vi "Host_PulseHistogram_OnlyLaser.vi"() -> ()   [LabVIEW 2012]
uses:
  <vilib>/FPGAPlugInAG/PXIe-7962R/niLvFpga_Open_PXIe-7962R.vi
  <vilib>/rvi/interface/common/dynamic/niFpgaDynamicAddResources.vi
  <vilib>/Utility/error.llb/Error Cluster From Error Code.vi
  <vilib>/rvi/errors/niLvFpgaAdjustHostInterfaceError.vi
  <vilib>/FPGAPlugInAG/Dynamic/niLvFpga_Close_Dynamic.vi
  <vilib>/rvi/interface/nirviOpenFPGA/nirviOpenFPGA.xnode
  FPGA Bitfiles/PulseHistogram_OnlyLaser_PXIe-7962R.lvbitx
  <vilib>/rvi/interface/nirviReadWriteControl/nirviReadWriteControl.xnode
  <vilib>/rvi/interface/nirviMethod/nirviMethod.xnode
  <vilib>/rvi/interface/nirviCloseFPGA/nirviCloseFPGA.xnode
  <vilib>/rvi/interface/Simulation/niFpgaSimulationCallBeginRW.vi
  NiFpgaLv.dll
  <vilib>/FPGAPlugInAG/Dynamic/niLvFpga_ReadFifo_Dynamic.vi
  <vilib>/rvi/errors/niLvFpgaMergeErrorWithErrorCode.vi
panel:
  out "Interflank intervals":i32[](graph)
  out "Loop counter":i32
  out "Waveform Graph":waveform(i16)(graph)
  out "Interloop FIFO timed out":bool
  out "Acq FIFO overflow":bool
  out "Interloop FIFO overflow":bool
  out "Reference pulse frequency":dbl format="%#_5p"
  out "Total sample count":u64
  out "Total reference pulse count":u64
  out "Reference pulse length histogram":T1(graph)
  out "Reference pulse period histogram":T1(graph)
  out "Sampling frequency":dbl format="%#_6p"
  out "Sampling interval":dbl format="%#_6p"
  in  "Onboard clock frequency":dbl=500000000.0 format="%#_6p"
  in  "Quit":bool
  # "Set clock before start!"
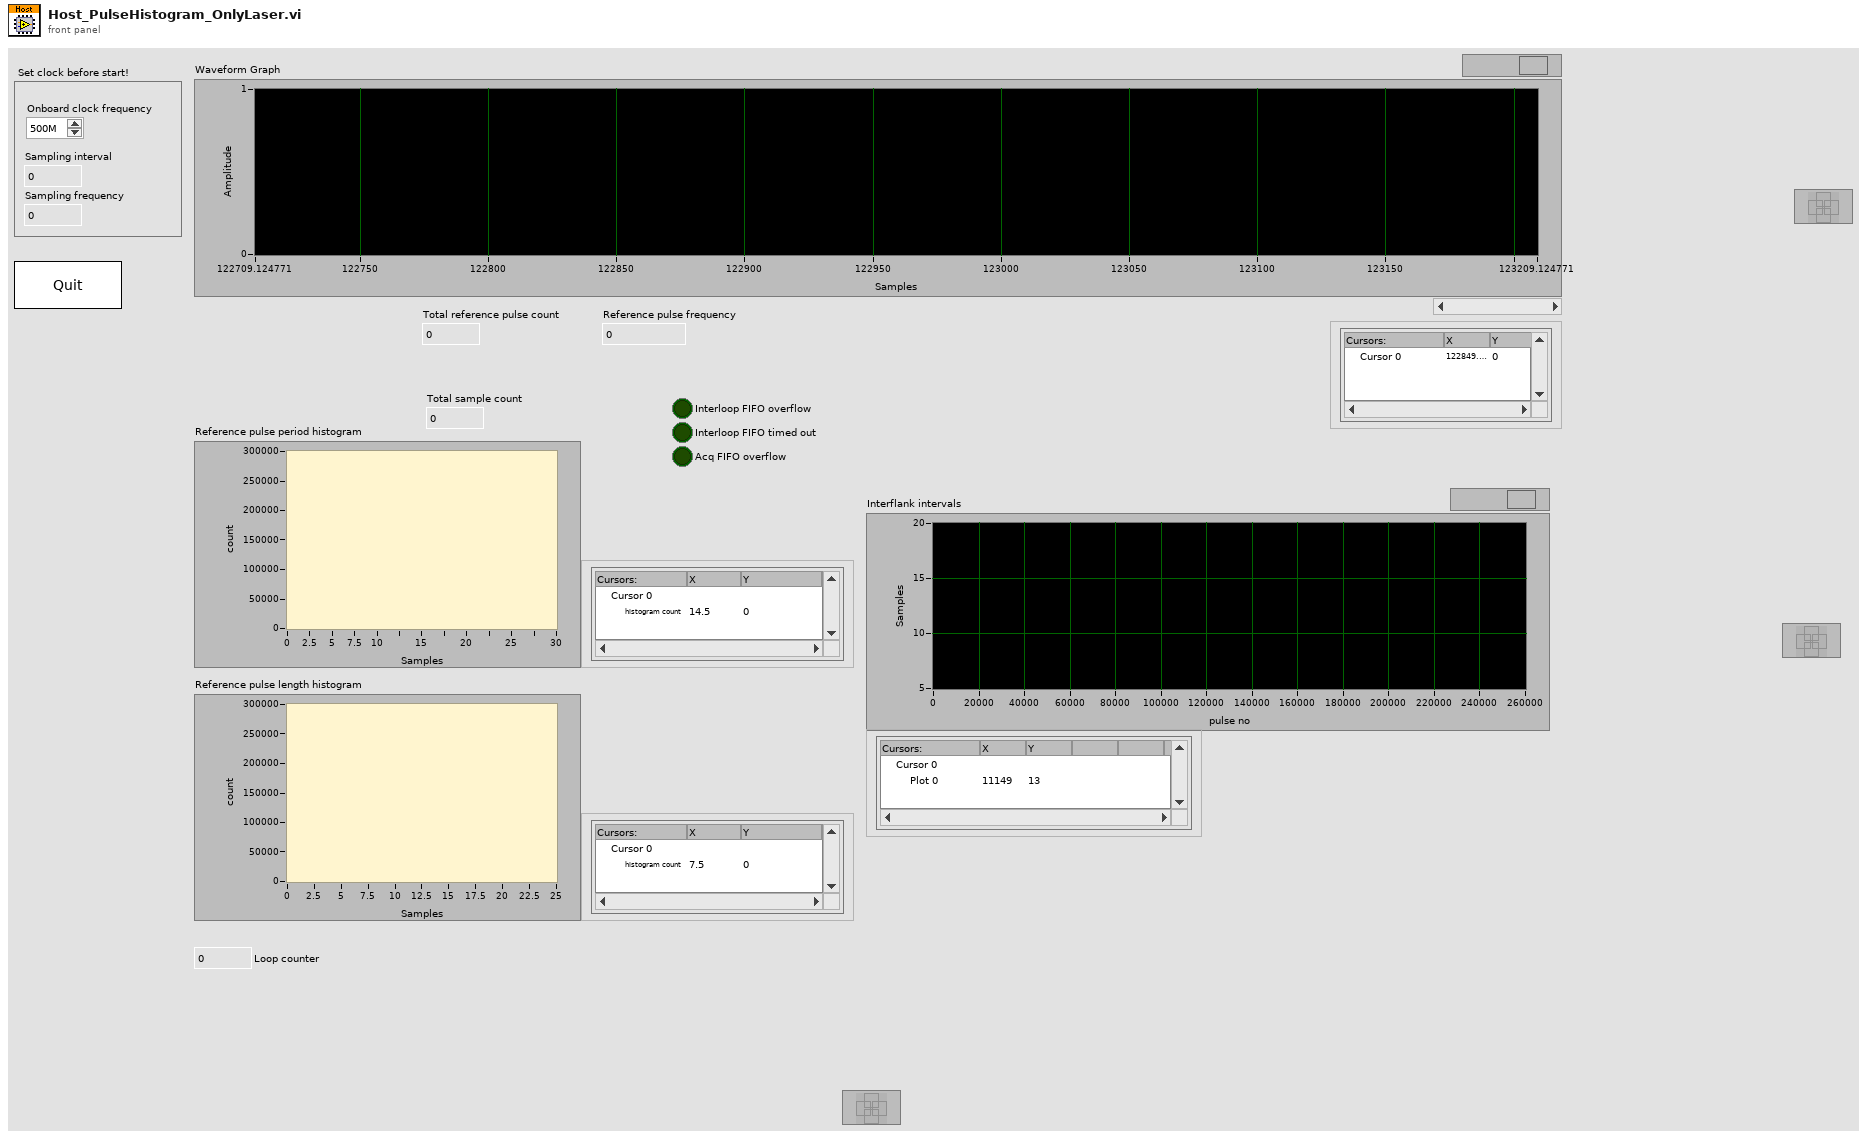
[diagram p1: front panel]
types:
  T1 = cluster{"X Values":dbl[], "Histogram: h(x)":i32[]}
  T2 = enum8{"Enabled", "Disabled", "Disabled and Grayed Out"}
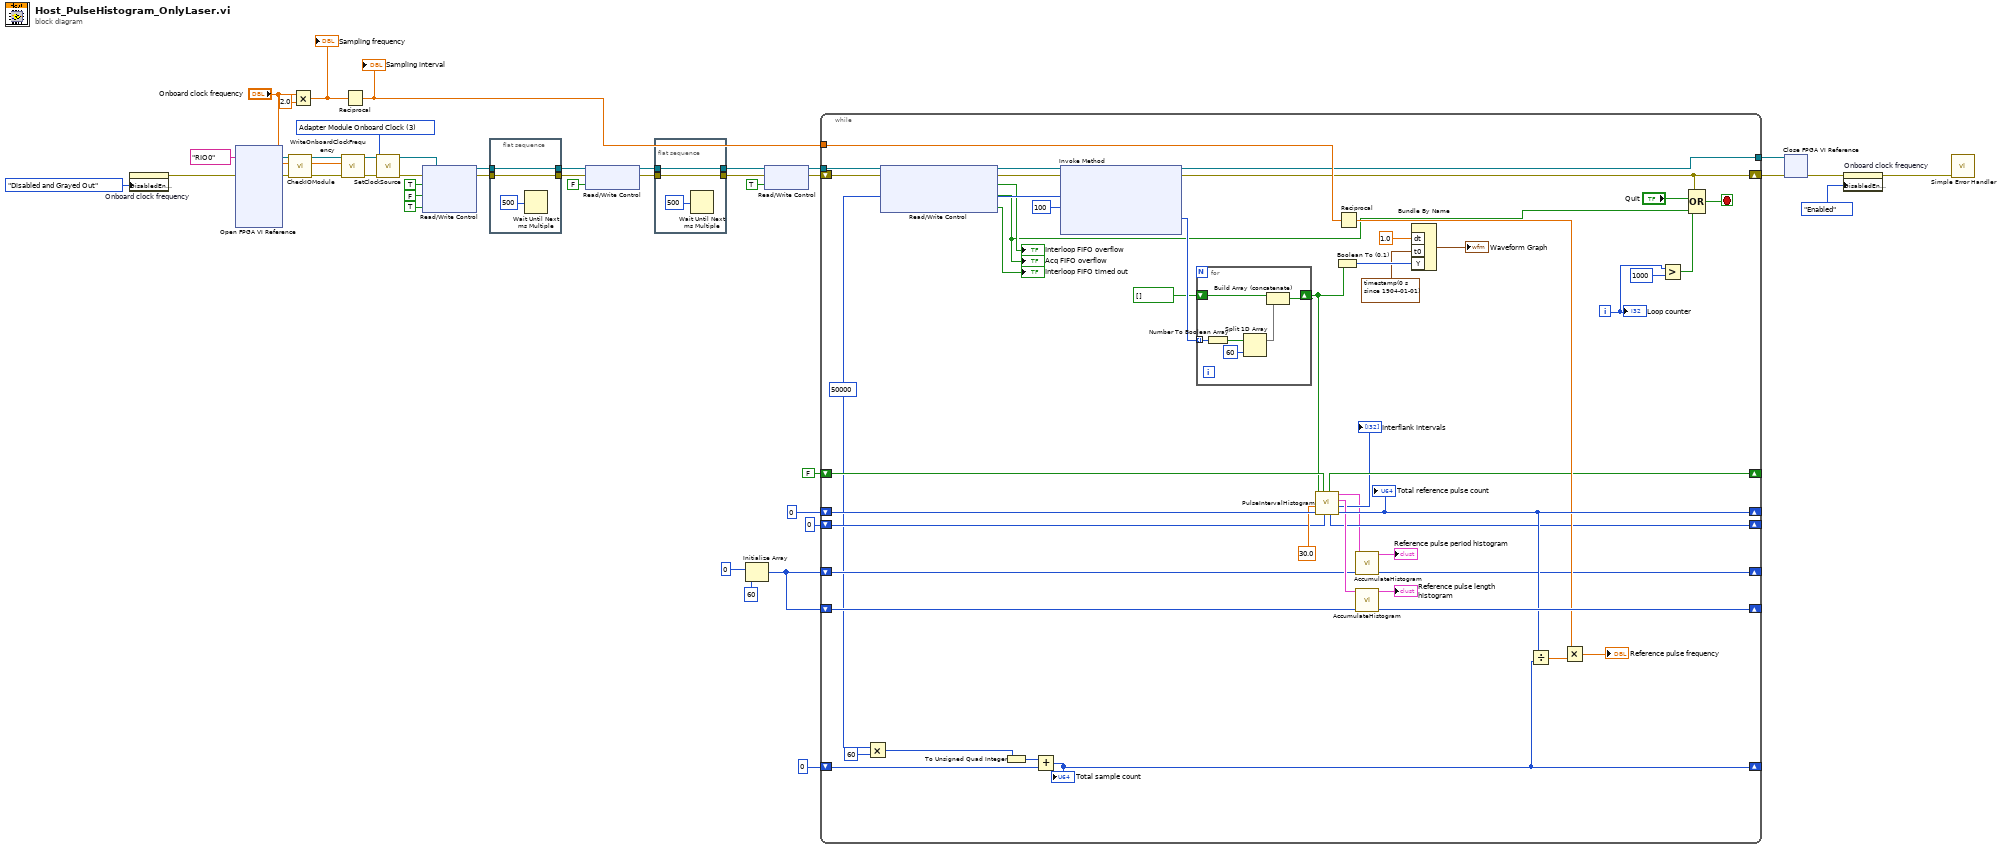
[diagram p0: block diagram]
diagram:
  w43 = u8 3 items=["Tristate"=0, "Sync Clock (PXIe only)"=2, "Adapter Module Onboard Clock"=3, "Strobe from Crosspoint Switch"=4, "Strobe Bypass"=5] ("Clock Source")
  n1 = property on="Onboard clock frequency" class="DigNum (strict)"("DisabledEnum"=T2."Disabled and Grayed Out" ("Disabled")) -> (error out=w27:errorcluster)  [unwired: 2 in, 1 out]
  n2 = xnode "Open FPGA VI Reference"("error in"=w27, "resource name"=tag "RIO0") -> ("FPGA VI Reference Out"=w7:refnum<k20>, "error out"=w6:errorcluster)
  n3 = call "CheckIOModule.vi"("error in (no error)"=w6, "FPGA VI Reference In"=w7) -> ("error out"=w37:errorcluster, "FPGA VI Reference Out"=w36:refnum<k20>)  [unwired: 8 in]
  n4 = Multiply(x="Onboard clock frequency", y=2.0) -> (x*y=w31:dbl)
  "Sampling frequency" <- w31
  n5 = call "WriteOnboardClockFrequency.vi"("error in (no error)"=w37, "Onboard clock frequency"="Onboard clock frequency", "FPGA VI Reference In"=w36) -> ("error out"=w35:errorcluster, "FPGA VI Reference Out"=w34:refnum<k20>)  [unwired: 7 in]
  n6 = Reciprocal(x=w31) -> (1/x=w30:dbl)
  "Sampling interval" <- w30
  n7 = call "SetClockSource.vi"("error in (no error)"=w35, "Clock Source"=w43, "FPGA VI Reference In"=w34) -> ("error out"=w41:errorcluster, "FPGA VI Reference Out"=w42:refnum<k20>)  [unwired: 7 in]
  n8 = xnode "Read/Write Control"("FPGA VI Reference In"=w42, "error in"=w41, "Commit"=TRUE, "Acq_Reset"=FALSE, "Acq_Reset"=TRUE) -> ("FPGA VI Reference Out"=w17:refnum<k20>, "error out"=w16:errorcluster)
  n9 = flat-sequence {
    tunnel: w17 -> [w44]
    tunnel: w16 -> [w45]
    tunnel: [w45] -> w14
    tunnel: [w44] -> w15
    frame #0 {
      n10 = Wait Until Next ms Multiple(millisecond multiple=u32 500) -> ()  [unwired: 1 out]
    }
  }
  n11 = xnode "Read/Write Control"("FPGA VI Reference In"=w15, "error in"=w14, "Acq_Reset"=FALSE) -> ("FPGA VI Reference Out"=w9:refnum<k20>, "error out"=w8:errorcluster)
  n12 = flat-sequence {
    tunnel: w9 -> [w47]
    tunnel: w8 -> [w48]
    tunnel: [w48] -> w4
    tunnel: [w47] -> w5
    frame #0 {
      n13 = Wait Until Next ms Multiple(millisecond multiple=u32 500) -> ()  [unwired: 1 out]
    }
  }
  n14 = Initialize Array(0, 60 ("dimension size")) -> (w19:i32[])
  n15 = xnode "Read/Write Control"("FPGA VI Reference In"=w5, "error in"=w4, "Acquire"=TRUE) -> ("FPGA VI Reference Out"=w3:refnum<k20>, "error out"=w2:errorcluster)
  n16 = while {
    tunnel: w3 -> [w54]
    tunnel: w30 -> [w82]
    shift-right: [w57] -> w29
    shift-left: w2 -> [w53]
    tunnel: [w58] -> w28
    shift-right: [w73] -> _
    shift-left: w19 -> [w63]
    shift-right: [w97] -> _
    shift-left: w19 -> [w96]
    shift-right: [w95] -> _
    shift-left: u64 0 ("Pulse count out") -> [w94]
    shift-right: [w69] -> _
    shift-left: u64 0 ("Pulse count out") -> [w93]
    shift-right: [w77] -> _
    shift-left: FALSE ("Last reference value out") -> [w76]
    shift-right: [w75] -> _
    shift-left: 0 ("Last rising flank out") -> [w74]
    i -> [w65]
    stop <- w72 stop-if-true
    w59 = u32 50000 ("Number of Elements")
    n17 = Multiply(x=w59, y=u32 60) -> (x*y=w84:u32)
    n18 = xnode "Read/Write Control"("FPGA VI Reference In"=w54, "error in"=w53) -> ("FPGA VI Reference Out"=w51:refnum<k20>, "error out"=w52:errorcluster, "Interloop FIFO overflow"=→"Interloop FIFO overflow":bool, "ToHostLaserFIFO overflow"=w50:bool, "Interloop FIFO timed out"=→"Interloop FIFO timed out":bool)
    "Acq FIFO overflow" <- w50
    n19 = To Unsigned Quad Integer(1:w84) -> (0:w83:u64)
    n20 = Add(x=w83, y=w93) -> (x+y=w69:u64)
    "Total sample count" <- w69
    n21 = xnode "Invoke Method"("FPGA VI Reference In"=w51, "error in"=w52, "Number of Elements"=w59, "Timeout (ms)"=100) -> ("FPGA VI Reference Out"=w58:refnum<k20>, "error out"=w57:errorcluster, "Data"=w86:u64[])  [unwired: 1 out]
    n22 = for {
      tunnel: w86 -> [w102] mode=indexing
      shift-right: [w100] -> w61
      shift-left: bool[] [] -> [w99]
      n23 = Number To Boolean Array(number=w102) -> (Boolean array=w103:bool[])
      n24 = Split 1D Array(array=w103, index=60) -> (first subarray=w98:bool[])  [unwired: 1 out]
      n25 = Build Array (concatenate)(w99, w98) -> (w100:bool[])
    }
    n26 = call "PulseIntervalHistogram.vi"("Last rising flank in"=w74, "Last reference value in"=w76, "Pulse count in"=w94, "No of SI bins"=30.0, "Binary array probe"=w61) -> ("Pulse count out"=w95:u64, "Interflank intervals out"=→"Interflank intervals":i32[], "Pulse length histogram"=w90:T1, "Pulse period histogram"=w64:T1, "Last rising flank out"=w75:i32, "Last reference value out"=w77:bool)  [unwired: 1 in]
    "Total reference pulse count" <- w95
    n27 = Boolean To (0,1)(Boolean=w61) -> (0, 1=w92:i16[])
    n28 = Reciprocal(x=w82) -> (1/x=w80:dbl)
    n29 = call "AccumulateHistogram.vi"("Array in"=w63, "Histogram graph in"=w64) -> ("Array out"=w73:i32[], "Histogram graph out"=→"Reference pulse period histogram":T1)  [unwired: 8 in]
    n30 = call "AccumulateHistogram.vi"("Array in"=w96, "Histogram graph in"=w90) -> ("Array out"=w97:i32[], "Histogram graph out"=→"Reference pulse length histogram":T1)  [unwired: 8 in]
    n31 = Bundle By Name("dt"=1.0, "t0"=timestamp(0 s since 1904-01-01), "Y"=w92) -> (→"Waveform Graph":waveform(i16))  [unwired: 1 in]
    n32 = Divide(x=w95, y=w69) -> (x/y=w87:dbl)
    n33 = Multiply(x=w80, y=w87) -> (x*y=→"Reference pulse frequency":dbl)
    n34 = Greater?(x=w65, y=1000) -> (0:w67:bool)
    n35 = Compound Arithmetic op=OR(w57, "Quit", w67, w50) -> (w72:bool)
    "Loop counter" <- w65
  }
  n36 = xnode "Close FPGA VI Reference"("FPGA VI Reference In"=w28, "error in"=w29) -> ("error out"=w25:errorcluster)
  n37 = property on="Onboard clock frequency" class="DigNum (strict)"(error in=w25, "DisabledEnum"=T2."Enabled" ("Disabled")) -> (error out=w21:errorcluster)  [unwired: 1 in, 1 out]
  n38 = call <vilib>:"Simple Error Handler.vi"("error in (no error)"=w21) -> ()  [unwired: 4 in, 5 out]
